vi "Write Nested Actor.vi"(10 "Nested Actor":refnum<class "Actor.lvclass">, 11 "Caller Endpoint in":refnum<class "Caller Endpoint.lvclass">) -> (3 "Caller Endpoint out":refnum<class "Caller Endpoint.lvclass">)   [LabVIEW 2020, in "Caller Endpoint.lvlib" / "Caller Endpoint.lvclass"]
doc: "Use this write accessor to set the actor to be launched by the Caller Endpoint. You must set this value prior to launching the actor."
uses:
  Caller Endpoint.lvclass
  <vilib>/ActorFramework/Actor/Actor.lvclass
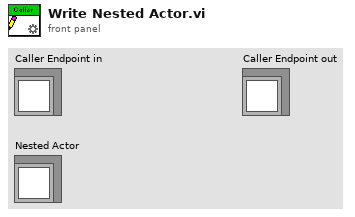
[diagram p1: front panel]
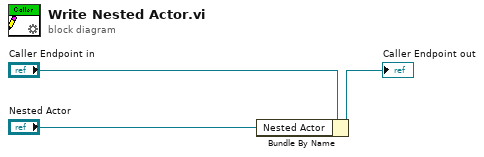
[diagram p0: block diagram]
diagram:
  n1 = Bundle By Name(cluster="Caller Endpoint in", "Nested Actor"="Nested Actor") -> (→"Caller Endpoint out":refnum<class "Caller Endpoint.lvclass">)
